vi "LabVIEW Options Updater.vi"() -> ()   [LabVIEW 2020]
uses:
  <vilib>/Utility/config.llb/Read Key (String).vi
  <resource>/dialog/lvconfig.llb/LV Config Write String.vi
  <resource>/dialog/lvconfig.llb/LV Config Write Numeric (I32).vi
  <resource>/dialog/lvconfig.llb/LV Config Write Boolean.vi
  <vilib>/Utility/config.llb/NI_LVConfig.lvlib
panel:
  out "values":string[](array[string])
  out "key names":string[](array[string])
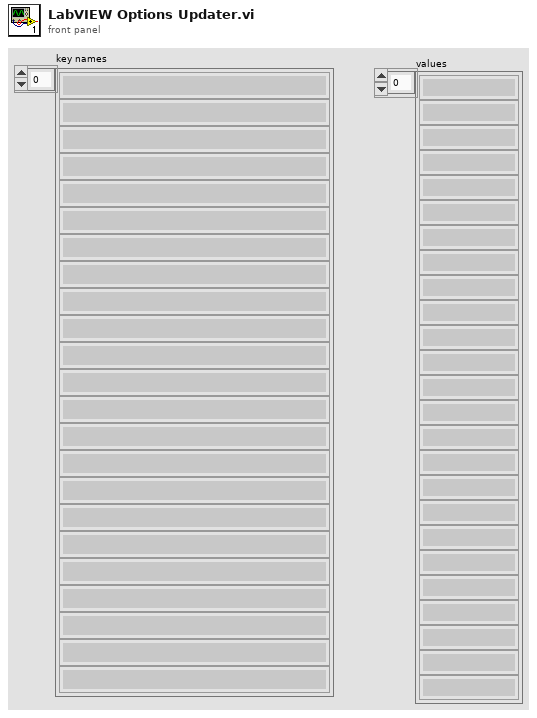
[diagram p1: front panel]
types:
  T1 = typedef "NI_LVConfig.lvlib/Config Data RefNum.ctl" = refnum<k1>
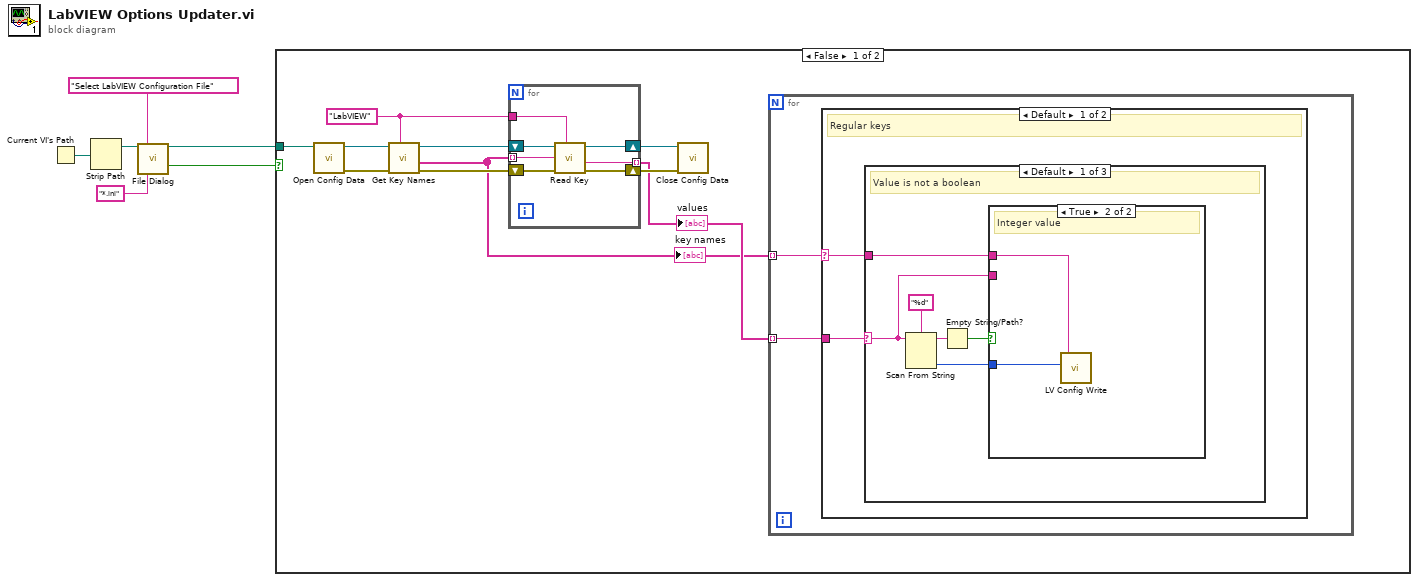
[diagram p0: block diagram]
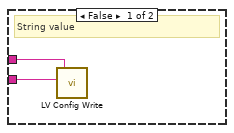
[diagram p2: hidden frame]
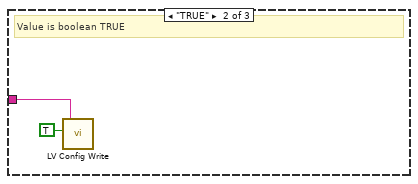
[diagram p3: hidden frame]
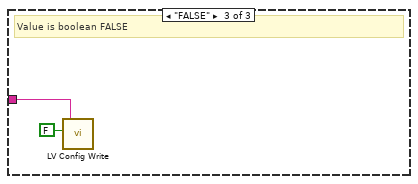
[diagram p4: hidden frame]
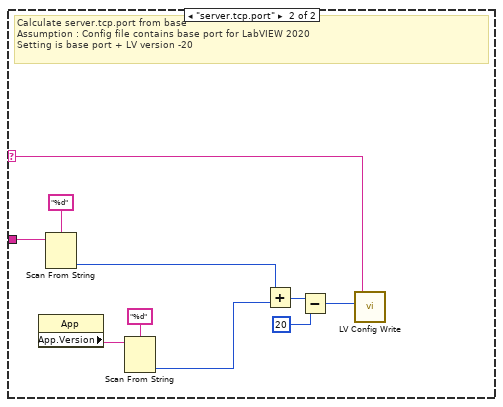
[diagram p5: hidden frame]
diagram:
  n1 = Current VI's Path() -> (path=w6:path)
  n2 = Strip Path(path=w6) -> (stripped path=w5:path)  [unwired: 1 out]
  n3 = call "File Dialog"("start path"=w5, "prompt"="Select LabVIEW Configuration File", "pattern (all files)"="*.ini" ("pattern")) -> ("selected path"=w1:path, "cancelled"=w2:bool)  [unwired: 9 in, 2 out]
  n4 = case shown="False" w2 {
    tunnel: w1 -> [w16 _]
    frame False {
      w9 = "LabVIEW" ("section")
      n5 = call <vilib>:"Open Config Data.vi"("configuration file path"=w16) -> ("error out"=w14:errorcluster, "refnum"=w15:T1)  [unwired: 8 in, 1 out]
      n6 = call <vilib>:"Get Key Names.vi"("section"=w9, "error in (no error)"=w14, "refnum"=w15) -> ("error out"=w13:errorcluster, "key names"=w7:string[], "refnum out"=w11:T1)  [unwired: 5 in, 1 out]
      "key names" <- w7
      n7 = for {
        shift-right: [w50] -> w12
        shift-left: w13 -> [w51]
        shift-right: [w48] -> w10
        shift-left: w11 -> [w49]
        tunnel: w7 -> [w45] mode=indexing
        tunnel: w9 -> [w47]
        tunnel: [w46] -> w8 mode=indexing
        n8 = call-poly <vilib>:"Read Key.vi"("section"=w47, "error in (no error)"=w51, "key"=w45, "refnum"=w49) -> ("error out"=w50:errorcluster, "value"=w46:string, "refnum out"=w48:T1)  [unwired: 4 in, 1 out]
      }
      "values" <- w8
      n9 = call <vilib>:"Close Config Data.vi"("error in (no error)"=w12, "refnum"=w10) -> ()  [unwired: 8 in, 2 out]
      n10 = for {
        tunnel: w7 -> [w17] mode=indexing
        tunnel: w8 -> [w18] mode=indexing
        n11 = case shown="Default" w17 {
          selector: w17 -> [w19 w39]
          tunnel: w18 -> [w20 w43]
          frame Default {
            # "Regular keys"
            n12 = case shown="Default" w20 {
              selector: w20 -> [w24 _ _]
              tunnel: w19 -> [w26 w31 w33]
              frame Default {
                # "Value is not a boolean"
                n13 = Scan From String(format string="%d", input string=w24) -> (remaining string=w23:string, output 1=w21:i32)  [unwired: 3 in, 2 out]
                n14 = Empty String/Path?(string/path=w23) -> (empty?=w22:bool)
                n15 = case shown="True" w22 {
                  tunnel: w24 -> [w28 _]
                  tunnel: w26 -> [w27 w30]
                  tunnel: w21 -> [_ w29]
                  frame False {
                    # "String value"
                    n16 = call-poly <resource>:"LV Config Write.vi"("value"=w28, "key"=w27) -> ()  [unwired: 5 in, 1 out]
                  }
                  frame True {
                    # "Integer value"
                    n17 = call-poly <resource>:"LV Config Write.vi"("value"=w29, "key"=w30) -> ()  [unwired: 5 in, 1 out]
                  }
                }
              }
              frame "TRUE" {
                # "Value is boolean TRUE"
                n18 = call-poly <resource>:"LV Config Write.vi"("value"=TRUE, "key"=w31) -> ()  [unwired: 5 in, 1 out]
              }
              frame "FALSE" {
                # "Value is boolean FALSE"
                n19 = call-poly <resource>:"LV Config Write.vi"("value"=FALSE, "key"=w33) -> ()  [unwired: 5 in, 1 out]
              }
            }
          }
          frame "server.tcp.port" {
            # "Calculate server.tcp.port from base\nAssumption : Config file contains base port for LabVIEW 2020\nSetting is base port + LV version -20"
            n20 = property class="App"() -> ("App.Version"=w37:string)  [unwired: 2 in, 2 out]
            n21 = Scan From String(format string="%d", input string=w43) -> (output 1=w40:i32)  [unwired: 3 in, 3 out]
            n22 = Scan From String(format string="%d", input string=w37) -> (output 1=w35:i32)  [unwired: 3 in, 3 out]
            n23 = Add(x=w40, y=w35) -> (x+y=w42:i32)
            n24 = Subtract(x=w42, y=20) -> (x-y=w38:i32)
            n25 = call-poly <resource>:"LV Config Write.vi"("value"=w38, "key"=w39) -> ()  [unwired: 5 in, 1 out]
          }
        }
      }
    }
    frame True {
    }
  }
